vi "Close RF Sessions.vi"(0 "RF Subsystem Session Provider in":refnum<class "RF Subsystem Session Provider.lvclass">, 5 "TSM Context":T1, 11 "error in":errorcluster) -> (4 "RF Subsystem Session Provider out":refnum<class "RF Subsystem Session Provider.lvclass">, 15 "error out":errorcluster)   [LabVIEW 2023, in "RFFixtureCharact.RMM.lvlib" / "RF Subsystem Session Provider.lvclass"]
uses:
  RF Subsystem Session Provider.lvclass
  <vilib>/NI_TestStand_SemiconductorModule/NI_TestStand_Semiconductor_Module.lvlibp/PinMap/General/SemiconductorModuleContext.ctl
  RF Subsystem Session Provider.lvclass/RF Subsystem Session Provider.ctl
  Common/RFCalAndFixtureCharact.Common.lvlib
  <vilib>/NI_TestStand_SemiconductorModule/NI_TestStand_Semiconductor_Module.lvlibp
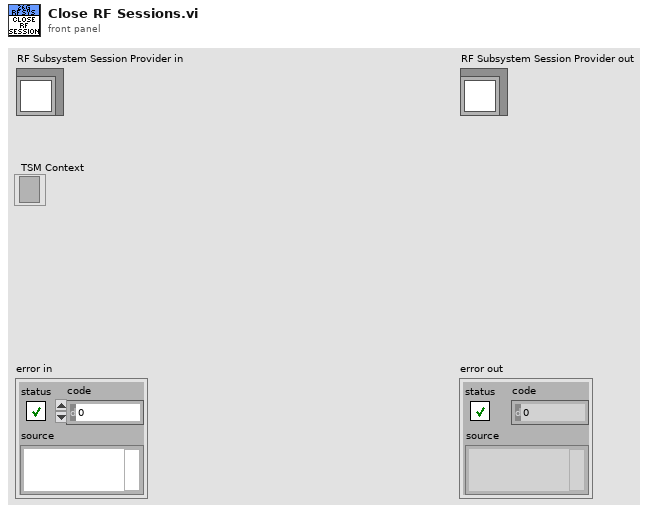
[diagram p1: front panel]
types:
  T1 = typedef "NI_TestStand_Semiconductor_Module.lvlibp/SemiconductorModuleContext.ctl" = refnum<k7>
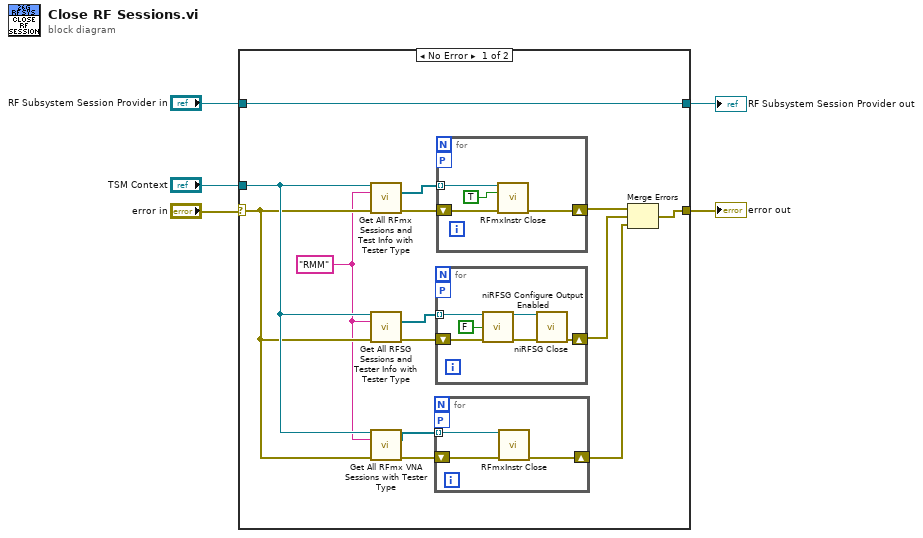
[diagram p0: block diagram]
diagram:
  n1 = case shown="No Error" "error in" {
    selector: "error in" -> [w10 w34]
    tunnel: [w12 w34] -> w2
    tunnel: "TSM Context" -> [w11 _]
    tunnel: "RF Subsystem Session Provider in" -> [w13 w33]
    tunnel: [w13 w33] -> w4
    frame No Error {
      w6 = "RMM"
      n2 = call "Get All RFmx Sessions and Test Info with Tester Type.vi"("TSM Context In"=w11, "Tester Type"=w6, "error in"=w10) -> ("RFmx Sessions"=w19:refnum<k21>[], "error out"=w17:errorcluster)  [unwired: 8 in, 3 out]
      n3 = call "Get All RFSG Sessions and Tester Info with Tester Type.vi"("TSM Context In"=w11, "Tester Type"=w6, "error in"=w10) -> ("RFSG Sessions"=w18:refnum<k15>[], "error out"=w16:errorcluster)  [unwired: 8 in, 3 out]
      n4 = call "Get All RFmx VNA Sessions with Tester Type.vi"("TSM Context In"=w11, "Tester Type"=w6, "error in"=w10) -> ("RFmx VNA Sessions"=w7:refnum<k21>[], "error out"=w9:errorcluster)  [unwired: 10 in, 1 out]
      n5 = for {
        workers-P: _ -> [_]
        shift-right: [w21] -> w8
        shift-left: w9 -> [w22]
        tunnel: w7 -> [w20] mode=indexing
        n6 = call <vilib>:"RFmxInstr Close.vi"("Instrument Handle In"=w20, "error in (no error)"=w22) -> ("error out"=w21:errorcluster)  [unwired: 13 in]
      }
      n7 = for {
        tunnel: w18 -> [w25] mode=indexing
        workers-P: _ -> [_]
        shift-right: [w28] -> w14
        shift-left: w16 -> [w27]
        n8 = call <instrlib>:"niRFSG Configure Output Enabled.vi"("instrument handle"=w25, "output enabled"=FALSE, "error in"=w27) -> ("instrument handle out"=w24:refnum<k15>, "error out"=w26:errorcluster)  [unwired: 11 in]
        n9 = call <instrlib>:"niRFSG Close.vi"("instrument handle"=w24, "error in"=w26) -> ("error out"=w28:errorcluster)  [unwired: 13 in]
      }
      n10 = for {
        tunnel: w19 -> [w32] mode=indexing
        workers-P: _ -> [_]
        shift-right: [w30] -> w15
        shift-left: w17 -> [w29]
        n11 = call <vilib>:"RFmxInstr Close.vi"("Instrument Handle In"=w32, "Force Destroy? (F)"=TRUE, "error in (no error)"=w29) -> ("error out"=w30:errorcluster)  [unwired: 12 in]
      }
      n12 = Merge Errors(w15, w14, w8) -> (w12:errorcluster)
    }
    frame Error {
    }
  }
  "error out" <- w2
  "RF Subsystem Session Provider out" <- w4
